vi "prueba Lester Roche y elmin mejia.vi"() -> ()   [LabVIEW 2011]
uses:
  Control 1.ctl
panel:
  out "Mayor a 35":bool[](array[boolean])
  out "Temperatura":i32[](array[slide]) scale=1.0..60.0
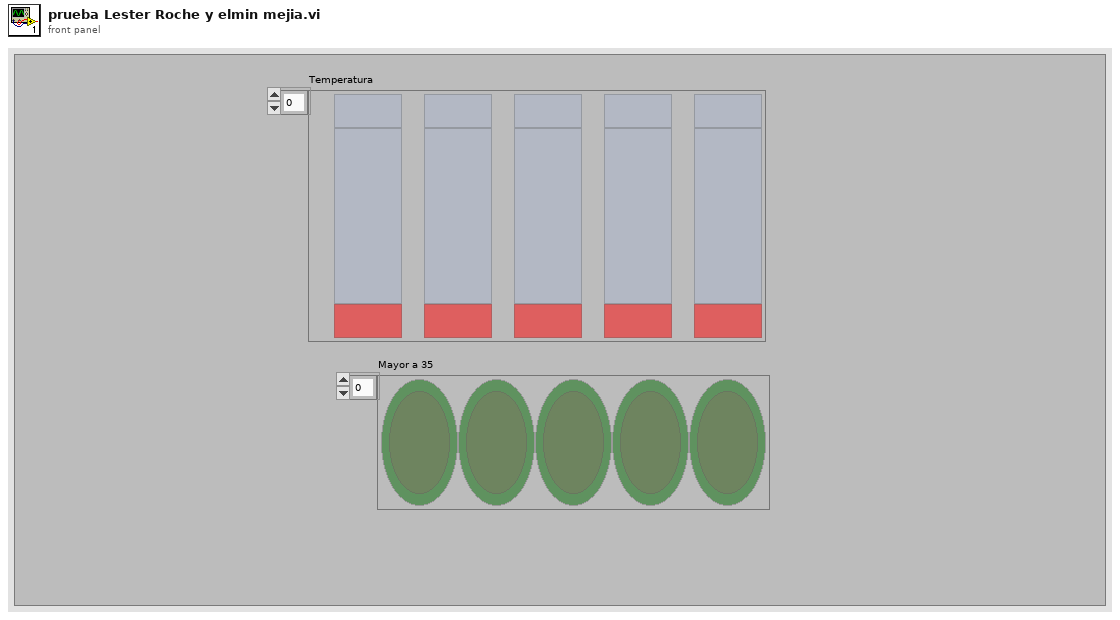
[diagram p1: front panel]
types:
  T1 = typedef "Control 1.ctl" = enum16{"Inicializar", "Rellenar arreglo de temp", "Leds mayor a 35", "finalizar"}
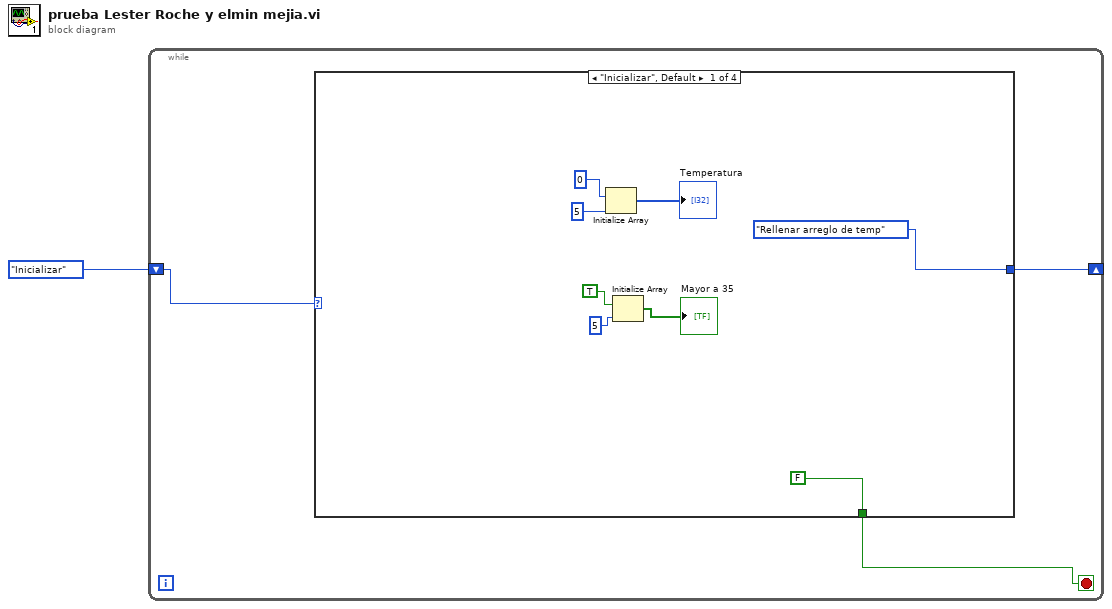
[diagram p0: block diagram]
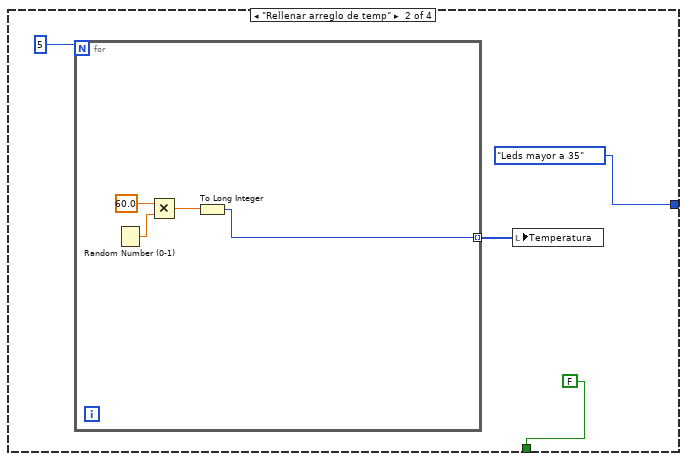
[diagram p2: hidden frame]
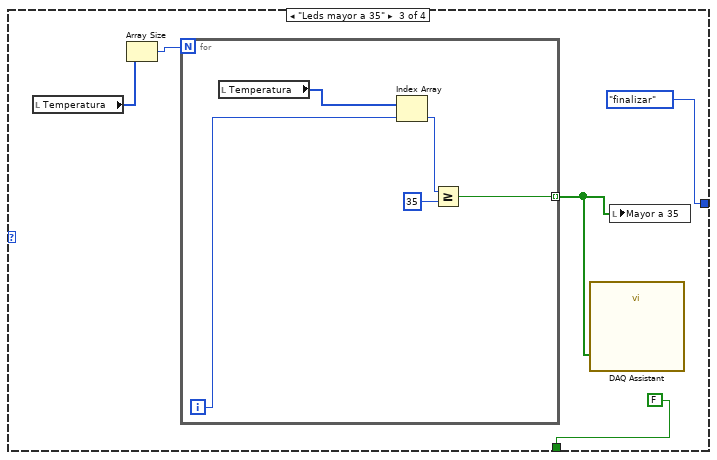
[diagram p3: hidden frame]
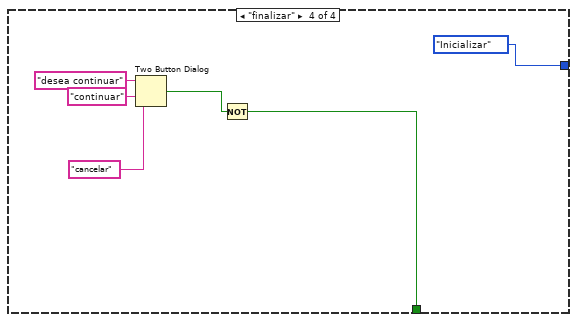
[diagram p4: hidden frame]
diagram:
  n1 = while {
    shift-right: [w3] -> _
    shift-left: Control_1."Inicializar" -> [w4]
    stop <- w2 stop-if-true
    n2 = case shown="\"Inicializar\", Default" w4 {
      tunnel: [Control_1."Rellenar arreglo de temp" Control_1."Leds mayor a 35" Control_1."finalizar" Control_1."Inicializar"] -> w3
      tunnel: [FALSE FALSE FALSE w31] -> w2
      frame "Inicializar", Default {
        n3 = Initialize Array(0, 5) -> (→"Temperatura":i32[])
        n4 = Initialize Array(TRUE, 5) -> (→"Mayor a 35":bool[])
      }
      frame "Rellenar arreglo de temp" {
        n5 = for {
          N: 5 -> [_]
          tunnel: [w17] -> w14 mode=indexing
          n6 = Random Number (0-1)() -> (number: 0 to 1=w19:dbl)
          n7 = Multiply(x=60.0, y=w19) -> (x*y=w18:dbl)
          n8 = To Long Integer(number=w18) -> (32bit integer=w17:i32)
        }
        n9 = local write "Temperatura"(w14) -> ()
      }
      frame "Leds mayor a 35" {
        n10 = local read "Temperatura"() -> (w24:i32[])
        n11 = Array Size(array=w24) -> (size(s)=w25:i32)
        n12 = for {
          N: w25 -> [_]
          tunnel: [w26] -> w21 mode=indexing
          i -> [w29]
          n13 = local read "Temperatura"() -> (w30:i32[])
          n14 = Index Array(array=w30, index=w29) -> (element=w28:i32)
          n15 = Greater Or Equal?(x=w28, y=35) -> (x >= y?=w26:bool)
        }
        n16 = call "DAQ Assistant"("data"=w21) -> ()  [unwired: 17 in, 2 out]
        n17 = local write "Mayor a 35"(w21) -> ()
      }
      frame "finalizar" {
        n18 = Two Button Dialog(message="desea continuar", 1:"cancelar" ("F button name (\"Cancel\")"), 2:"continuar" ("T button name (\"OK\")")) -> (T button?=w32:bool)
        n19 = Not(x=w32) -> (.not. x?=w31:bool)
      }
    }
  }
